vi "Tarea Semaforo.vi"() -> ()   [LabVIEW 2010]
panel:
  in  "stop":bool
  out "verde":bool
  out "amarillo":bool
  out "rojo":bool
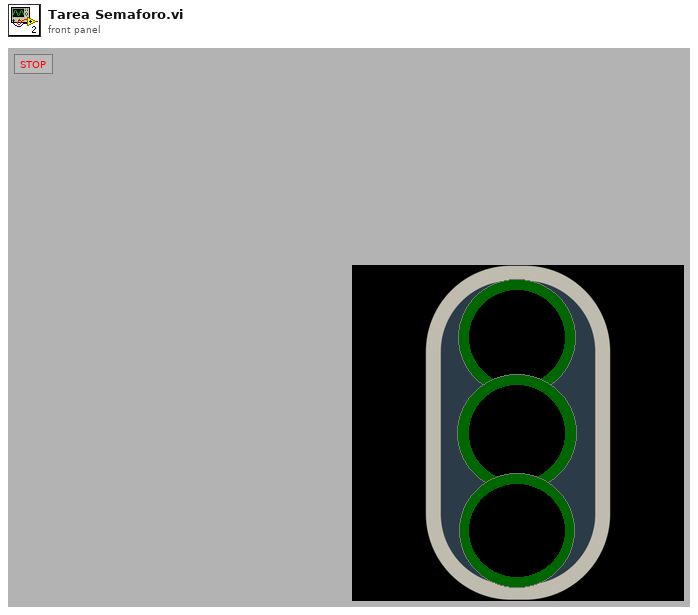
[diagram p1: front panel]
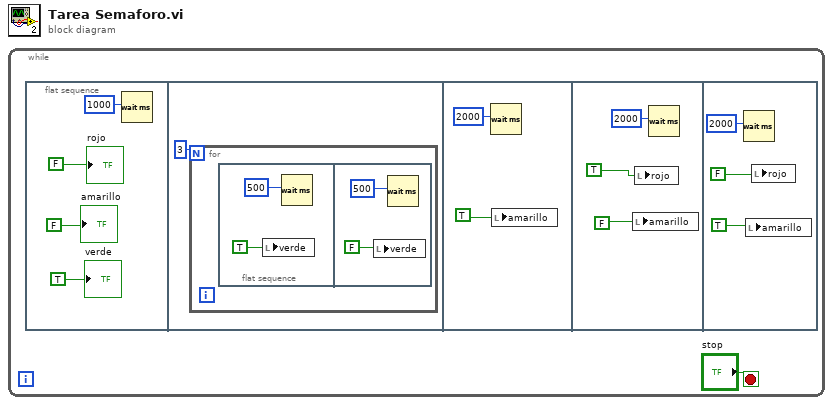
[diagram p0: block diagram]
diagram:
  n1 = while {
    stop <- "stop" stop-if-true
    n2 = flat-sequence {
      frame #0 {
        n3 = Wait (ms)(milliseconds to wait=1000) -> ()  [unwired: 1 out]
        "verde" <- TRUE
        "amarillo" <- FALSE
        "rojo" <- FALSE
      }
      frame #1 {
        n4 = for {
          N: 3 -> [_]
          n5 = flat-sequence {
            frame #0 {
              n6 = local write "verde"(TRUE) -> ()
              n7 = Wait (ms)(milliseconds to wait=500) -> ()  [unwired: 1 out]
            }
            frame #1 {
              n8 = local write "verde"(FALSE) -> ()
              n9 = Wait (ms)(milliseconds to wait=500) -> ()  [unwired: 1 out]
            }
          }
        }
      }
      frame #2 {
        n10 = Wait (ms)(milliseconds to wait=2000) -> ()  [unwired: 1 out]
        n11 = local write "amarillo"(TRUE) -> ()
      }
      frame #3 {
        n12 = local write "amarillo"(FALSE) -> ()
        n13 = local write "rojo"(TRUE) -> ()
        n14 = Wait (ms)(milliseconds to wait=2000) -> ()  [unwired: 1 out]
      }
      frame #4 {
        n15 = Wait (ms)(milliseconds to wait=2000) -> ()  [unwired: 1 out]
        n16 = local write "amarillo"(TRUE) -> ()
        n17 = local write "rojo"(FALSE) -> ()
      }
    }
  }
